vi "Sequence Dialog.vi"(8 "error in (no error)":errorcluster, 11 "Sequence Conditions In":T2 {"Sequence Controller"."Valve" items=["None", "LOX Press", "LOX Purge", "LOX Vent", "LOX Iso", "LOX Main", "LOX Bleed", "*open*", "Fuel Press", "Fuel Purge", "Fuel Vent", "Fuel Iso", "Fuel Main", "Film Cooling", "*open*", "Ignition"]}) -> (0 "error out":errorcluster, 1 "Cancelled?":bool=TRUE, 2 "UI Refresh Needed?":bool, 3 "Sequence Conditions Out":T2 {"Sequence Controller"."Valve" items=["None", "LOX Press", "LOX Purge", "LOX Vent", "LOX Iso", "LOX Main", "LOX Bleed", "*open*", "Fuel Press", "Fuel Purge", "Fuel Vent", "Fuel Iso", "Fuel Main", "Film Cooling", "*open*", "Ignition"]})   [LabVIEW 2024]
doc: "Dialog for selecting user specified settings."
uses:
  Sequence Structure.ctl
  Sequence Sorter.vi/f9d632dd-b722-4371-9ee4-7d5e9a90ae0c.vi
  Sequence Sorter.vi/ce6833b3-19ad-4906-ad44-d4b5e8c938f3.vi
  Sequence Sorter.vi/5cf53b88-c2f6-46cc-83b6-9af652960e03.vi
  Sequence Sorter.vi/165fc907-ca4c-4944-97e7-f355a83536ad.vi
  <vilib>/Utility/xml.llb/Write to XML File(string).vi
  <vilib>/Comparison/Equal/Equal Functor/Equal Functor.lvclass
  <vilib>/Comparison/Less/Less Functor/Less Functor.lvclass
panel:
  in  "Save as Preset":bool
  in  "Sequence Duration":dbl
  in  "Sequence Delay":dbl
  in  "Load Preset":bool
  in  "Sequence Controller":T1(array[cluster]) {"Valve" items=["None", "LOX Press", "LOX Purge", "LOX Vent", "LOX Iso", "LOX Main", "LOX Bleed", "*open*", "Fuel Press", "Fuel Purge", "Fuel Vent", "Fuel Iso", "Fuel Main", "Film Cooling", "*open*", "Ignition", "Trigger"]}
  in  "Cancel Button":bool
  in  "OK Button":bool
  # "Sequence Conditions"
  # "sec"
  # "sec"
  # "Non visible portion of dialog (needed for connector pane)."
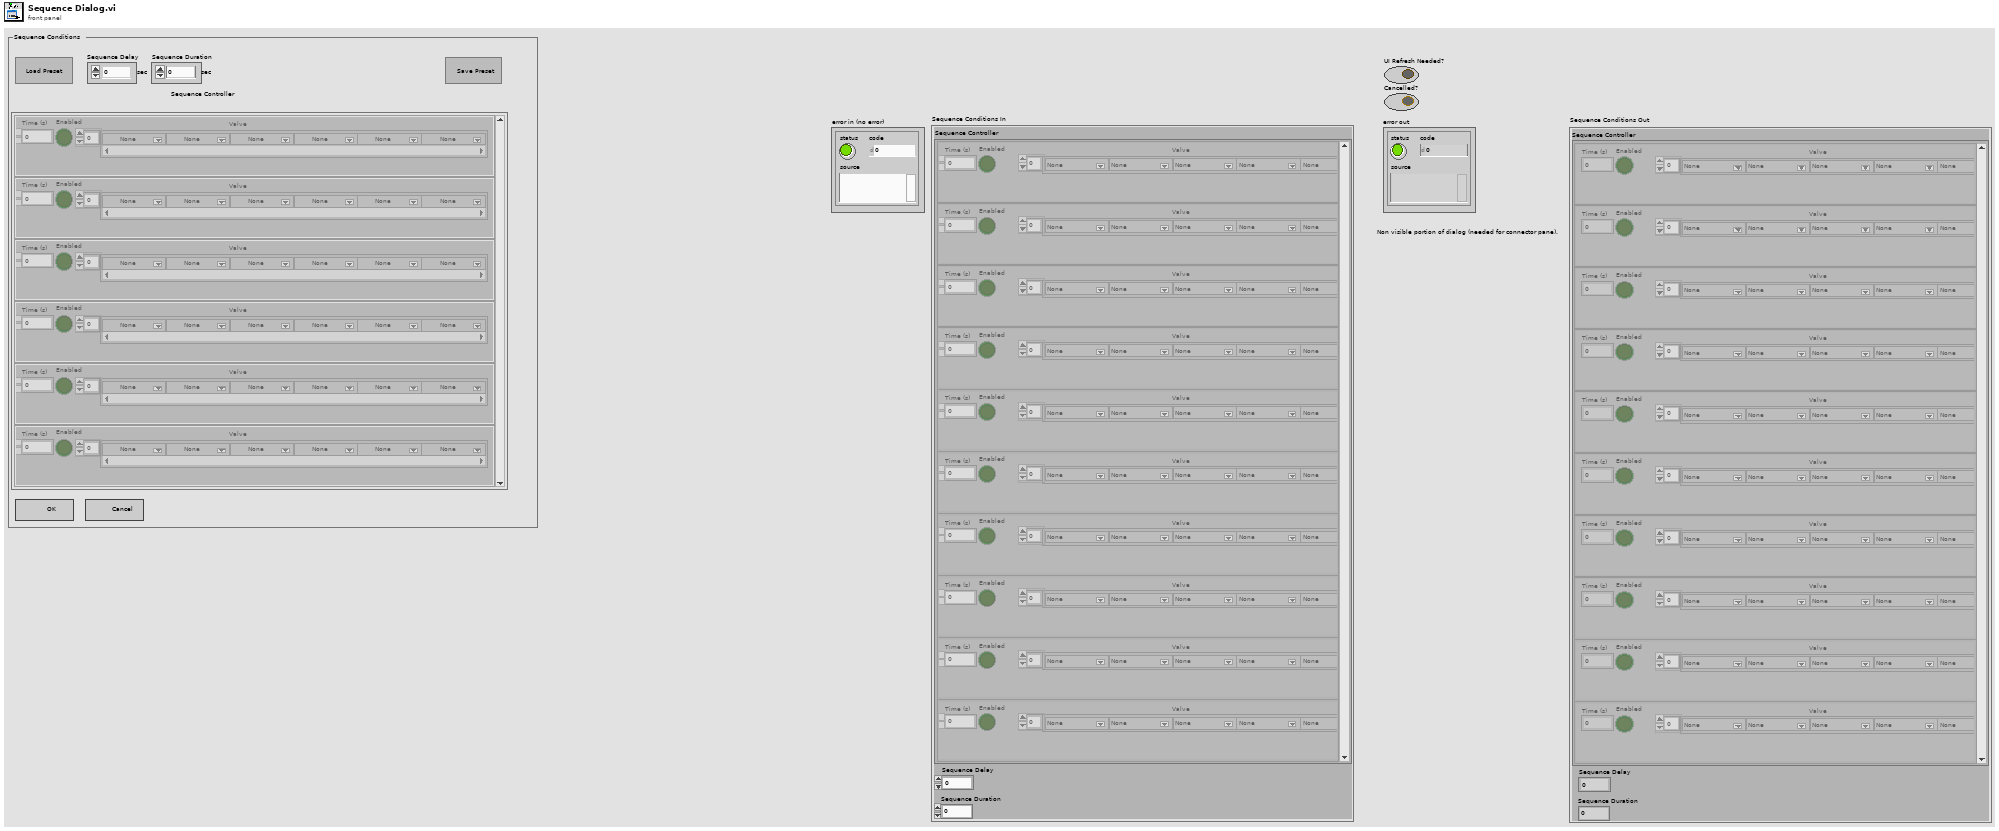
[diagram p1: front panel]
types:
  T1 = cluster{"Time (s)":dbl, "Enabled":bool, "Valve":u16[]}[]
  T2 = typedef "Sequence Structure.ctl" = cluster{"Sequence Controller":cluster{"Time (s)":dbl, "Enabled":bool, "Valve":u16[]}[], "Sequence Delay":dbl, "Sequence Duration":dbl}
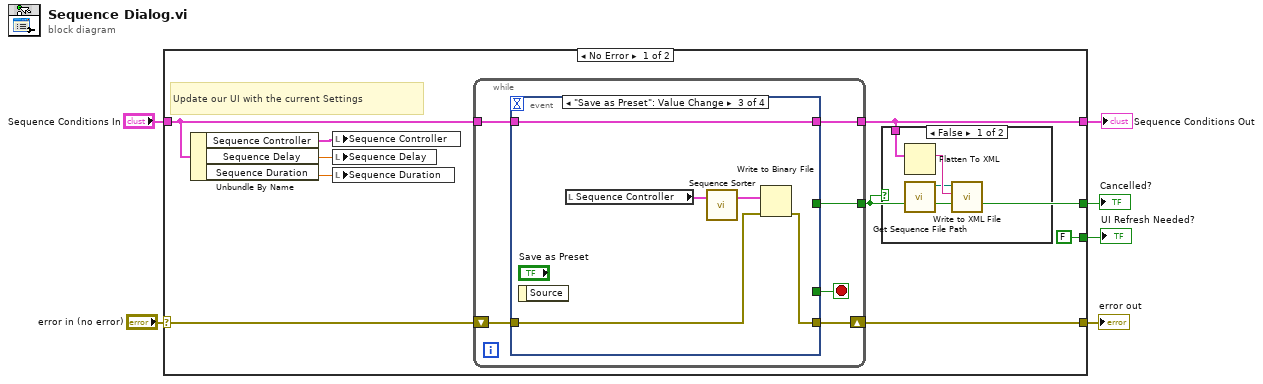
[diagram p0: block diagram]
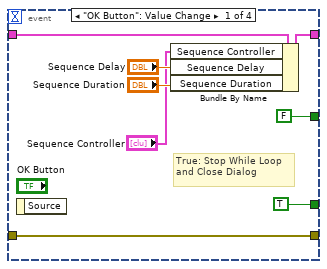
[diagram p3: hidden frame]
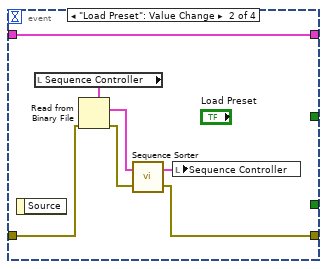
[diagram p4: hidden frame]
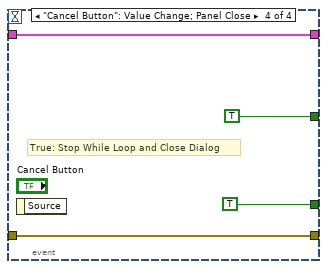
[diagram p5: hidden frame]
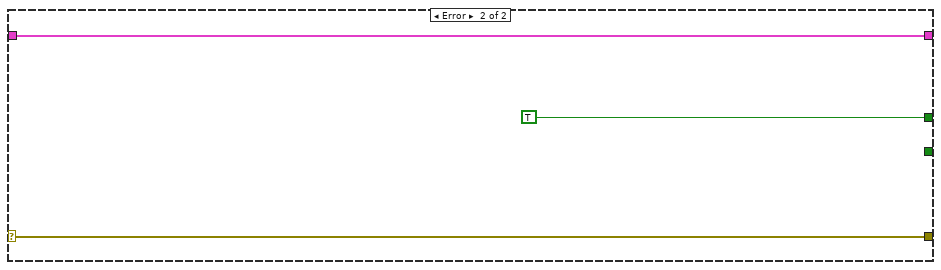
[diagram p6: hidden frame]
diagram:
  n1 = case shown="No Error" "error in (no error)" {
    selector: "error in (no error)" -> [w8 w51]
    tunnel: [w7 w51] -> w6
    tunnel: "Sequence Conditions In" -> [w14 w50]
    tunnel: [w9 w50] -> w1
    tunnel: [FALSE ("UI Refresh Needed?") _] -> w5
    tunnel: [w10 TRUE ("UI Refresh Needed?")] -> w4
    frame No Error {
      # "Update our UI with the current Settings"
      n2 = Unbundle By Name(w14) -> ("Sequence Controller"=w13:T1, "Sequence Delay"=w12:dbl, "Sequence Duration"=w11:dbl)
      n3 = local write "Sequence Controller"(w13) -> ()
      n4 = local write "Sequence Delay"(w12) -> ()
      n5 = local write "Sequence Duration"(w11) -> ()
      n6 = while {
        tunnel: [w24] -> w10
        tunnel: [w23] -> w9
        tunnel: w14 -> [w22]
        shift-right: [w19] -> w7
        shift-left: w8 -> [w20]
        stop <- w21 stop-if-true
        n7 = event shown="[2] \"Save as Preset\": Value Change" {
          selector: _ -> [_ _ _ _]
          dyn-events: _ -> [_ _ _ _]
          timeout: _ -> [_ _ _ _]
          tunnel: [w29 w39 w44 w48] -> w23
          tunnel: w22 -> [w30 w39 w44 w48]
          tunnel: [FALSE ("UI Refresh Needed?") _ _ TRUE ("UI Refresh Needed?")] -> w24
          tunnel: [TRUE _ _ TRUE] -> w21
          tunnel: w20 -> [w25 w33 w41 w45]
          tunnel: [w25 w35 w40 w45] -> w19
          event "OK Button": Value Change {
            # "True: Stop While Loop \nand Close Dialog"
            n8 = event-data() -> ()  [unwired: 1 in, 1 out]
            n9 = Bundle By Name(cluster=w30, "Sequence Controller"="Sequence Controller", "Sequence Delay"="Sequence Delay", "Sequence Duration"="Sequence Duration") -> (w29:T2)
          }
          event "Load Preset": Value Change {
            n10 = event-data() -> ()  [unwired: 1 in, 1 out]
            n11 = local read "Sequence Controller"() -> (w37:T1)
            n12 = Read from Binary File(5:w37, 8:w33) -> (0:w34:errorcluster, 2:w38:T1)  [unwired: 4 in, 2 out]
            n13 = call "Sequence Sorter.vi"("error in"=w34, "sequence in"=w38) -> ("error out"=w35:errorcluster, "sequence out"=w36:T1)
            n14 = local write "Sequence Controller"(w36) -> ()
          }
          event "Save as Preset": Value Change {
            n15 = event-data() -> ()  [unwired: 1 in, 1 out]
            n16 = local read "Sequence Controller"() -> (w43:T1)
            n17 = call "Sequence Sorter.vi"("sequence in"=w43) -> ("sequence out"=w42:T1)  [unwired: 1 in, 1 out]
            n18 = Write to Binary File(data=w42, error in=w41) -> (error out=w40:errorcluster)  [unwired: 4 in, 2 out]
          }
          event "Cancel Button": Value Change; Panel Close {
            # "True: Stop While Loop and Close Dialog"
            n19 = event-data() -> ()  [unwired: 1 in, 1 out]
          }
        }
      }
      n20 = case shown="False" w10 {
        tunnel: w9 -> [w18 _]
        frame False {
          n21 = Flatten To XML(6:w18) -> (2:w17:string)
          n22 = call "Get Sequence File Path.vi"() -> ("XML File Path"=w16:path)  [unwired: 10 in, 1 out]
          n23 = call-poly <vilib>:"Write to XML File.vi"("XML Input"=w17, "XML File Path"=w16) -> ()  [unwired: 7 in, 3 out]
        }
        frame True {
        }
      }
    }
    frame Error {
    }
  }
  "UI Refresh Needed?" <- w5
  "error out" <- w6
  "Cancelled?" <- w4
  "Sequence Conditions Out" <- w1
